vi "MB ICPCON Param Read timeouts.vi"(8 "error in (no error)":errorcluster, 11 "Param Reference in":T1) -> (0 "error out":errorcluster, 1 "timeouts":T2[](array[typedef]), 3 "Param Reference out":T1)   [LabVIEW 2021, in "ICPCON_Param.lvlib"]
uses:
  ICPCON_Param.lvlib
  ICPCON Param.ctl
  Eth timeouts.ctl
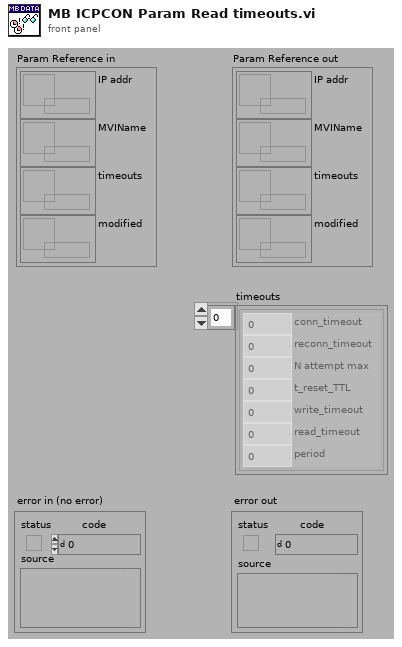
[diagram p1: front panel]
types:
  T1 = typedef "ICPCON_Param.lvlib/ICPCON Param.ctl" = cluster{"IP addr":refnum<data-value>, "MVIName":refnum<data-value>, "timeouts":refnum<data-value>, "modified":refnum<data-value>}
  T2 = typedef "ICPCON_Param.lvlib/Eth timeouts.ctl" = cluster{"conn_timeout":i32, "reconn_timeout":i32, "N attempt max":i32, "t_reset_TTL":i32, "write_timeout":i32, "read_timeout":i32, "period":i32}
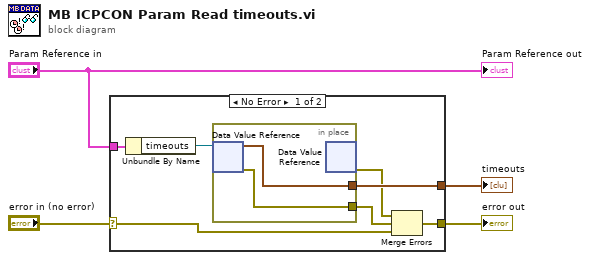
[diagram p0: block diagram]
diagram:
  n1 = case shown="No Error" "error in (no error)" {
    selector: "error in (no error)" -> [w5 w14]
    tunnel: [w9 w14] -> w4
    tunnel: [w11 _] -> w3
    tunnel: "Param Reference in" -> [w10 _]
    frame No Error {
      n2 = Unbundle By Name(w10) -> ("timeouts"=w6:refnum<data-value>)
      n3 = in-place {
        in-place-border: [w12] -> w11
        in-place-border: [w13] -> w7
        n4 = in-place-dvr #1(w6) -> (w12:T2[], w13:errorcluster)
        n5 = in-place-dvr #1() -> (w8:errorcluster)  [unwired: 1 in, 1 out]
      }
      n6 = Merge Errors(w8, w7, w5) -> (w9:errorcluster)
    }
    frame Error {
    }
  }
  "error out" <- w4
  "timeouts" <- w3
  "Param Reference out" <- "Param Reference in"
